vi "Update Busy Time.vi"(8 "error in (no error)":errorcluster, 11 "GenBus_Load_Calculator in":refnum<class "CANBus_Load_Calculator.lvclass">) -> (0 "error out":errorcluster, 3 "GenBus_Load_Calculator out":refnum<class "CANBus_Load_Calculator.lvclass">)   [LabVIEW 2018, in "NI-XNET Monitor Engine.lvlib" / "XNET-Bus-Load-Calculator.lvlib" / "CANBus_Load_Calculator.lvclass"]
uses:
  CANBus_Load_Calculator.lvclass
  typedefs/ToCalculator_Data.ctl
  CANBus_Load_Calculator.lvclass/CANBus_Load_Calculator.ctl
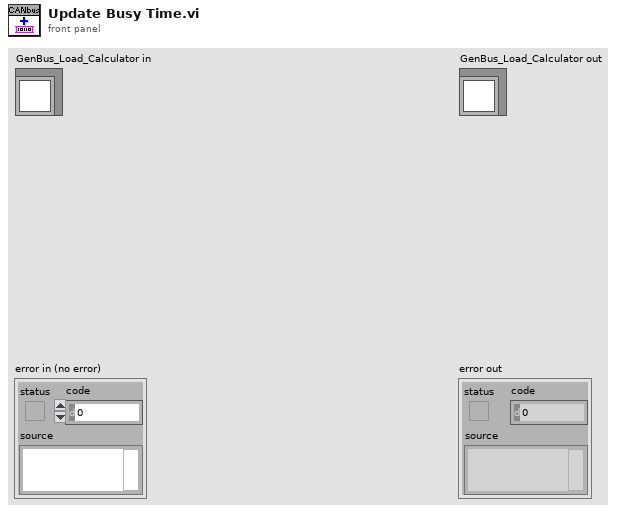
[diagram p1: front panel]
types:
  T1 = typedef "NI-XNET Monitor Engine.lvlib/XNET-Bus-Load-Calculator.lvlib/CANBus_Load_Calculator.lvclass/ToCalculator_Data.ctl" = cluster{"Stop":bool, "Bus Busy Time (us)":u64}
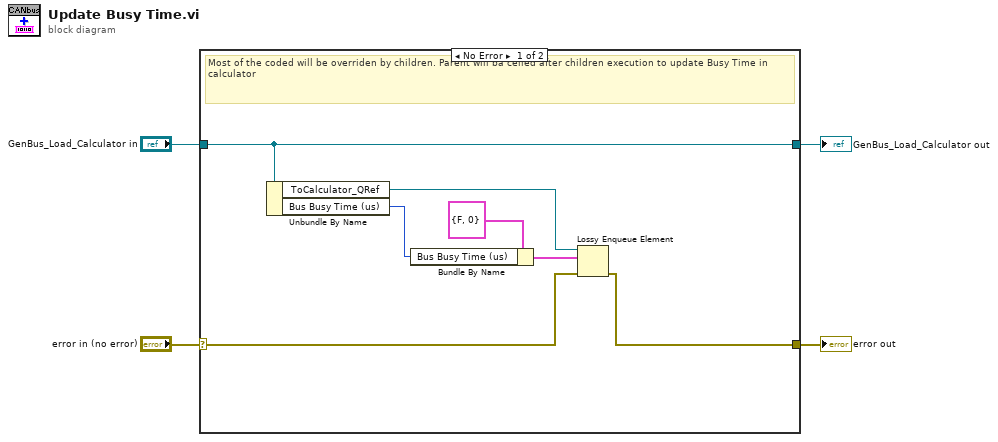
[diagram p0: block diagram]
diagram:
  n1 = case shown="No Error" "error in (no error)" {
    selector: "error in (no error)" -> [w9 w13]
    tunnel: [w8 w13] -> w3
    tunnel: [w11 w12] -> w1
    tunnel: "GenBus_Load_Calculator in" -> [w11 w12]
    frame No Error {
      # "Most of the coded will be overriden by children. Parent will ba celled after children execution to update Busy Time in calculator"
      n2 = Unbundle By Name(w11) -> ("ToCalculator_QRef"=w10:refnum<queue>, "Bus Busy Time (us)"=w5:u64)
      n3 = Bundle By Name(cluster=T1 {"Stop"=FALSE, "Bus Busy Time (us)"=0} ("element"), "Bus Busy Time (us)"=w5) -> (w6:T1)
      n4 = Lossy Enqueue Element(queue=w10, element=w6, error in (no error)=w9) -> (error out=w8:errorcluster)  [unwired: 3 out]
    }
    frame Error {
    }
  }
  "error out" <- w3
  "GenBus_Load_Calculator out" <- w1
